vi "GetWindowHandle.vi"(8 "error in (no error)":errorcluster, 11 "Window in":refnum<class "Window.lvclass">) -> (0 "error out":errorcluster, 2 "SDL_Window *":i64, 3 "Window out":refnum<class "Window.lvclass">)   [LabVIEW 2024, in "GLF.lvlib" / "Window.lvclass"]
uses:
  Window.lvclass
  Window.lvclass/Window.ctl
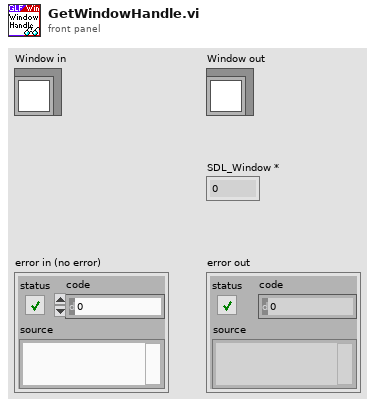
[diagram p1: front panel]
types:
  T1 = typedef "GLF.lvlib/Window.lvclass/DVR--cluster.ctl" = cluster{"SDL_Window *":i64}
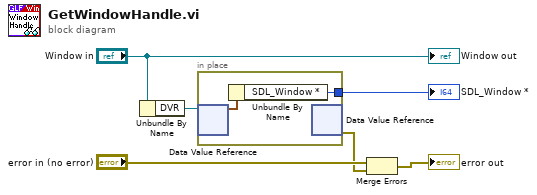
[diagram p0: block diagram]
diagram:
  n1 = Unbundle By Name("Window in") -> ("DVR"=w2:refnum<data-value>)
  n2 = in-place {
    in-place-border: [w8] -> w5
    n3 = in-place-dvr #1(w2) -> (w7:T1)  [unwired: 1 out]
    n4 = Unbundle By Name(w7) -> ("SDL_Window *"=w8:i64)
    n5 = in-place-dvr #1() -> (w1:errorcluster)  [unwired: 1 in, 1 out]
  }
  "SDL_Window *" <- w5
  n6 = Merge Errors("error in (no error)", w1) -> (→"error out":errorcluster)
  "Window out" <- "Window in"
